vi "Write Experiment Description (cluster).vi"(8 "error in (no error)":errorcluster, 10 "Experiment Description":T1={"User"="", "Device"="", "Device Path"=path "", "Device Description"="", "Experiment Path"=path "", "Experiment Description"="", "Instrument"=enum."MNK", "Instruments"=[], "Sweep"=[{"key"="OFF", "value"=variant}, {"key"="OFF", "value"=variant}, {"key"="OFF", "value"=variant}, {"key"="OFF", "value"=variant}]}, 11 "Control Experiment in":refnum<class "Control Experiment.lvclass">) -> (0 "error out":errorcluster, 3 "Control Experiment out":refnum<class "Control Experiment.lvclass">)   [LabVIEW 2019, in "Control Experiment.lvclass"]
uses:
  Control Experiment.lvclass
  Typedefs/Experiment Description--cluster.ctl
  Typedefs/Instrument--enum.ctl
  Typedefs/Instruments--cluster.ctl
  Typedefs/Instrument Types--enum.ctl
  Control Experiment.lvclass/Control Experiment.ctl
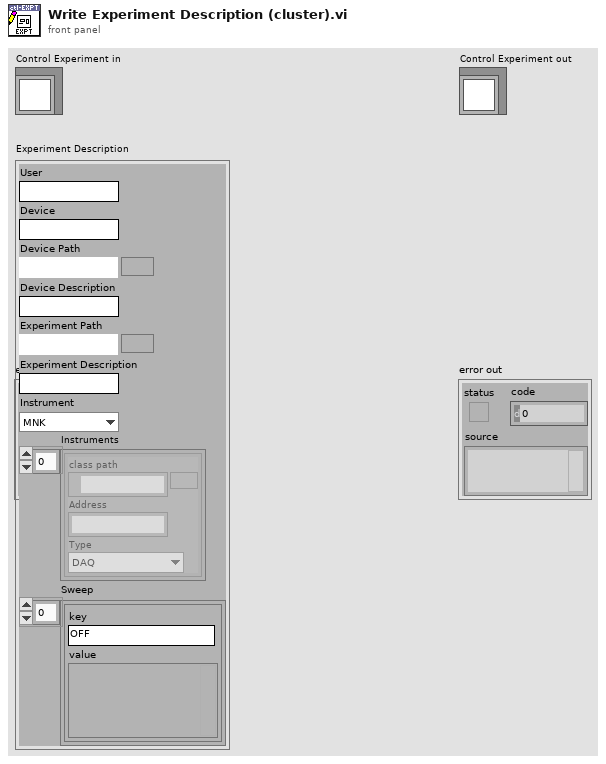
[diagram p1: front panel]
types:
  T1 = typedef "Control Experiment.lvclass/Experiment Description--cluster.ctl" = cluster{"User":string, "Device":string, "Device Path":path, "Device Description":string, "Experiment Path":path, "Experiment Description":string, "Instrument":T2, "Instruments":T3[], "Sweep":cluster{"key":string, "value":variant}[]}
  T2 = typedef "Control Experiment.lvclass/Instrument--enum.ctl" = enum16{"----- AFM -----", "AGILENT", "CYPHER", "JEOL", "MFP3D", "Omicron VT XA", "----- EBL -----", "Gemini2", "Omicron", "eLine", "----- Cryostat -----", "CF900", "DR200", "MNK", "PPMS (simulated)", "PPMS 1", "PPMS 2", "PPMS 3", "----- Optics -----", "THz 1 (Element 2/Montana)", "THz 2 (Tsunami/OptiCool)"}
  T3 = typedef "Control Experiment.lvclass/Instruments--cluster.ctl" = cluster{"class path":path, "Address":string, "Type":T4}
  T4 = typedef "Control Experiment.lvclass/Instrument Types--enum.ctl" = enum16{"DAQ", "Amplifier", "Temperature", "Magnet", "Rotator", "Level", "Capacitance", "Delay Line", "Strain Cell", "VNA", "Source"}
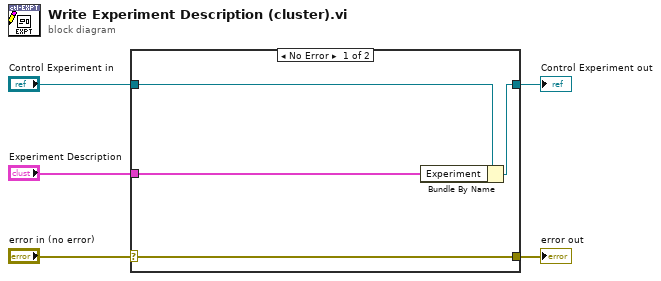
[diagram p0: block diagram]
diagram:
  n1 = case shown="No Error" "error in (no error)" {
    selector: "error in (no error)" -> [w9 w10]
    tunnel: [w9 w10] -> w4
    tunnel: [w7 w11] -> w2
    tunnel: "Control Experiment in" -> [w8 w11]
    tunnel: "Experiment Description" -> [w6 _]
    frame No Error {
      n2 = Bundle By Name(cluster=w8, "Experiment"=w6) -> (w7:refnum<class "Control Experiment.lvclass">)
    }
    frame Error {
    }
  }
  "error out" <- w4
  "Control Experiment out" <- w2
